vi "Play Sound Effx.vi"(7 "event":enum16{"Play", "Stop"}(ring), 8 "error in (no error)":errorcluster, 9 "path":path, 10 "Sound Effect Off":T1, 11 "Sounds In":T3(array[cluster]) {"Task ID" format="%.0x"}) -> (0 "error out":errorcluster, 3 "Sounds Out":T3(array[cluster]) {"Task ID" format="%.0x"})   [LabVIEW 2021]
uses:
  Typedefs/Sound Effects.ctl
  <vilib>/sound2/lvsound2.llb/Sound Output Task ID.ctl
  <vilib>/sound2/lvsound2.llb/Sound Output Set Volume (Single).vi
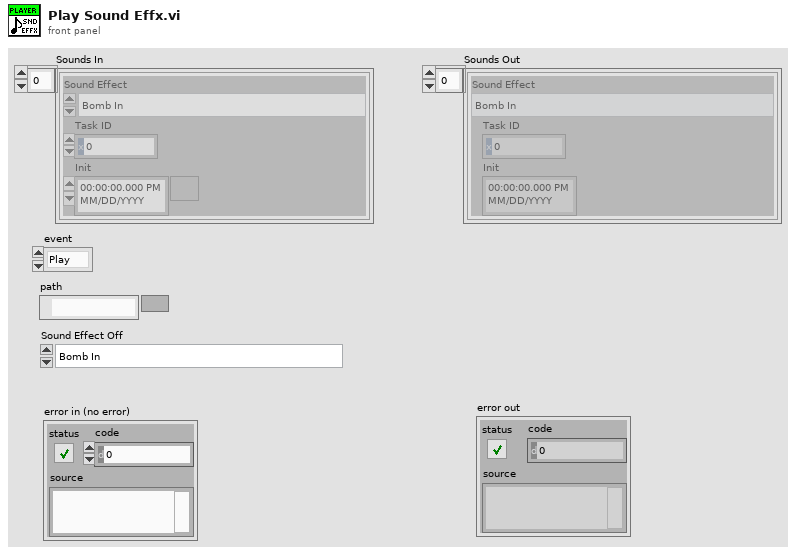
[diagram p1: front panel]
types:
  T1 = typedef "Sound Effects.ctl" = enum16{"Bomb In", "Bomb Out", "Bomb Touched", "Game Over", "Victory", "Eat", "10 Fruits", "Eat2", "Eat3", "Eat4", "MaxShield", "Shield", "10p", "Grape In", "Grape Out", "20p", "30p", "40p", "50p", "60p", "70p", "80p", "90p", "100p", "All shields cracked", "Mouse In", "Mouse Out", "Mouse Eaten", "Grape Eaten", "States Recover", "Broken Shield", "Bonus", "Happy Time", "explode", "Game over musica", "Back Music", "Shield Catch", "Evil lough", "Cricket In", "Cricket eaten", "Lets Go", "Jump1", "Jump2", "Jump3", "Unstoppable", "Troll Music", "winner"}
  T2 = typedef "Sound Output Task ID.ctl" = u32
  T3 = cluster{"Sound Effect":T1, "Task ID":T2, "Init":timestamp}[]
  T4 = cluster{"Sound Effect":T1, "Task ID":T2, "Init":timestamp}
  T5 = cluster{"Sound Effect Off":T1, "task ID":T2, "seconds since 1Jan1904":timestamp}
  T6 = cluster{"Sound Effect Off":T1, "task ID":T2, "seconds since 1Jan1904":timestamp}[]
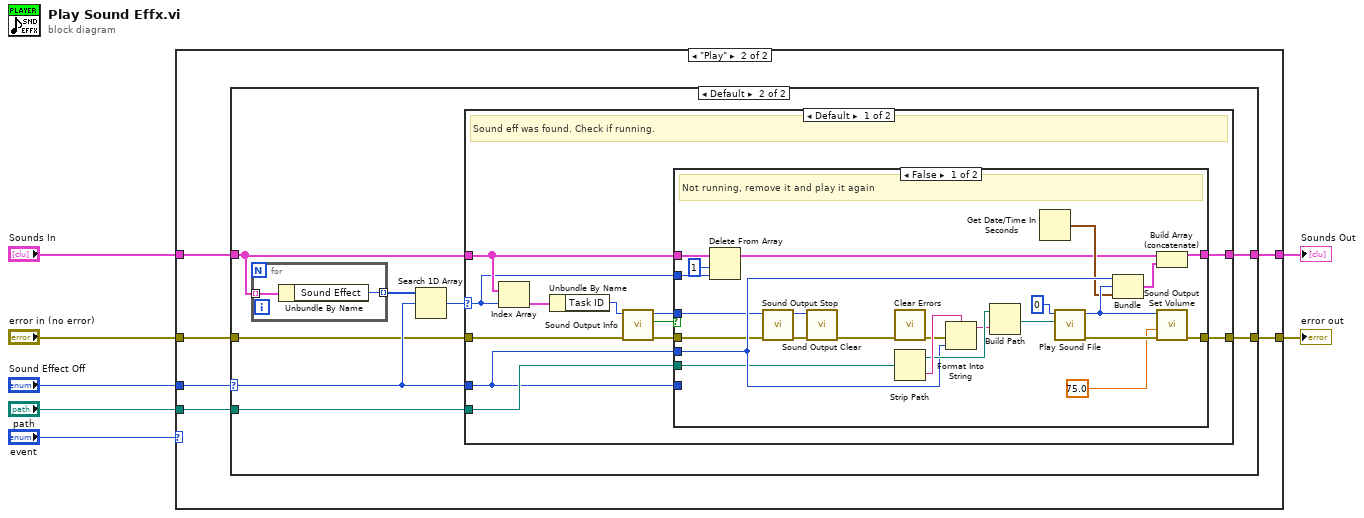
[diagram p0: block diagram]
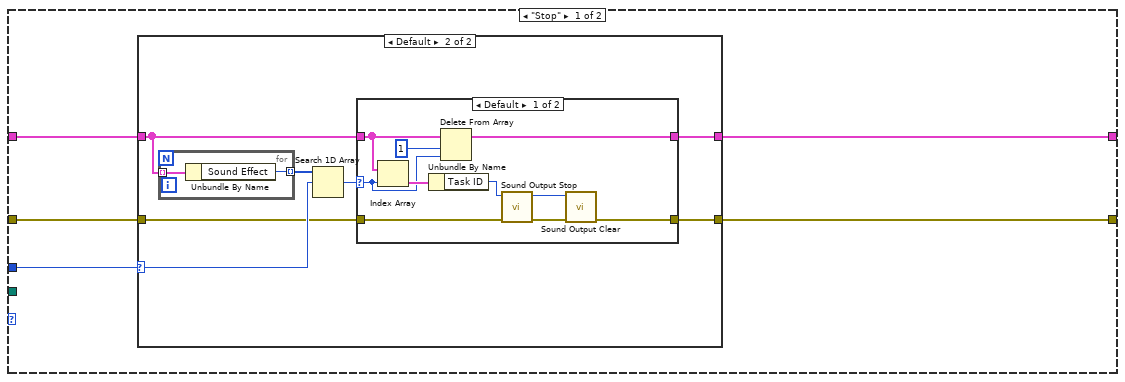
[diagram p2: hidden frame]
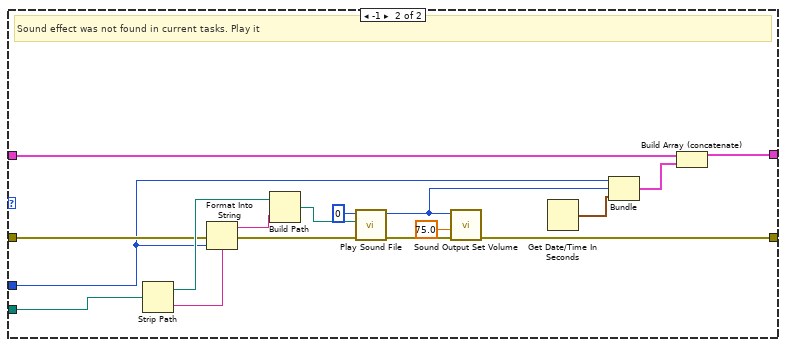
[diagram p7: hidden frame]
diagram:
  n1 = case shown="\"Play\"" "event" {
    tunnel: [w12 w41] -> w7
    tunnel: "Sounds In" -> [w11 w40]
    tunnel: "Sound Effect Off" -> [w10 w39]
    tunnel: "path" -> [_ w38]
    tunnel: [w8 w37] -> w1
    tunnel: "error in (no error)" -> [w9 w36]
    frame "Stop" {
      n2 = case shown="Default" w10 {
        selector: w10 -> [_ w21]
        tunnel: w11 -> [w14 w18]
        tunnel: [w14 w17] -> w12
        tunnel: w9 -> [w13 w16]
        tunnel: [w13 w15] -> w8
        frame "Back Music" {
        }
        frame Default {
          n3 = for {
            tunnel: w18 -> [w35] mode=indexing
            tunnel: [w34] -> w20 mode=indexing
            n4 = Unbundle By Name(w35) -> ("Sound Effect"=w34:T1)
          }
          n5 = Search 1D Array(1D array=w20, element=w21) -> (index of element=w19:i32)  [unwired: 1 in]
          n6 = case shown="Default" w19 {
            selector: w19 -> [w25 _]
            tunnel: w18 -> [w27 w33]
            tunnel: [w24 w33] -> w17
            tunnel: w16 -> [w23 w32]
            tunnel: [w22 w32] -> w15
            frame Default {
              n7 = Index Array(array=w27, index=w25) -> (element=w31:T4)
              n8 = Unbundle By Name(w31) -> ("Task ID"=w30:T2)
              n9 = Delete From Array(array=w27, length=1, index=w25) -> (array with subset deleted=w24:T3)  [unwired: 1 out]
              n10 = call <vilib>:"Sound Output Stop.vi"("error in (no error)"=w23, "task ID"=w30) -> ("error out"=w28:errorcluster, "task ID out"=w29:T2)  [unwired: 8 in]
              n11 = call <vilib>:"Sound Output Clear.vi"("error in (no error)"=w28, "task ID"=w29) -> ("error out"=w22:errorcluster)  [unwired: 9 in]
            }
            frame -1 {
            }
          }
        }
      }
    }
    frame "Play" {
      n12 = case shown="Default" w39 {
        selector: w39 -> [_ w47]
        tunnel: w40 -> [w43 w49]
        tunnel: [w43 w48] -> w41
        tunnel: w38 -> [_ w46]
        tunnel: [w42 w45] -> w37
        tunnel: w36 -> [w42 w44]
        frame "Back Music" {
        }
        frame Default {
          n13 = for {
            tunnel: w49 -> [w108] mode=indexing
            tunnel: [w107] -> w51 mode=indexing
            n14 = Unbundle By Name(w108) -> ("Sound Effect"=w107:T1)
          }
          n15 = Search 1D Array(1D array=w51, element=w47) -> (index of element=w50:i32)  [unwired: 1 in]
          n16 = case shown="Default" w50 {
            selector: w50 -> [w52 _]
            tunnel: w49 -> [w60 w98]
            tunnel: [w59 w97] -> w48
            tunnel: w47 -> [w53 w92]
            tunnel: w46 -> [w56 w96]
            tunnel: [w55 w95] -> w45
            tunnel: w44 -> [w54 w94]
            frame Default {
              # "Sound eff was found. Check if running."
              n17 = Index Array(array=w60, index=w52) -> (element=w63:T4)
              n18 = Unbundle By Name(w63) -> ("Task ID"=w62:T2)
              n19 = call <vilib>:"Sound Output Info.vi"("error in (no error)"=w54, "task ID"=w62) -> ("error out"=w57:errorcluster, "is playing?"=w61:bool, "task ID out"=w58:T2)  [unwired: 6 in, 1 out]
              n20 = case shown="False" w61 {
                tunnel: w60 -> [w80 w89]
                tunnel: [w79 w89] -> w59
                tunnel: w58 -> [w73 _]
                tunnel: w57 -> [w72 w88]
                tunnel: w53 -> [w77 _]
                tunnel: w56 -> [w76 _]
                tunnel: [w70 w88] -> w55
                tunnel: w53 -> [_ _]
                tunnel: w52 -> [w65 _]
                frame False {
                  # "Not running, remove it and play it again"
                  n21 = Delete From Array(array=w80, length=1, index=w65) -> (array with subset deleted=w66:T3)  [unwired: 1 out]
                  n22 = call <vilib>:"Sound Output Stop.vi"("error in (no error)"=w72, "task ID"=w73) -> ("error out"=w74:errorcluster, "task ID out"=w75:T2)  [unwired: 8 in]
                  n23 = call <vilib>:"Sound Output Clear.vi"("error in (no error)"=w74, "task ID"=w75) -> ("error out"=w71:errorcluster)  [unwired: 9 in]
                  n24 = call <vilib>:"Clear Errors.vi"("error in (no error)"=w71) -> ("error out"=w69:errorcluster)  [unwired: 5 in, 1 out]
                  n25 = Strip Path(path=w76) -> (stripped path=w84:path, name=w85:string)
                  n26 = Format Into String(format string=w85, error in=w69, w77) -> (resulting string=w83:string)  [unwired: 1 in, 1 out]
                  n27 = Build Path(base path=w84, name or relative path=w83) -> (appended path=w82:path)
                  n28 = Get Date/Time In Seconds() -> (seconds since 1Jan1904=w67:timestamp)
                  n29 = call <vilib>:"Play Sound File.vi"("path"=w82, "device ID"=u32 0) -> ("error out"=w86:errorcluster, "task ID"=w81:T2)  [unwired: 8 in]
                  n30 = Bundle("Sound Effect Off"=w77, "task ID"=w81, "seconds since 1Jan1904"=w67) -> (w78:T5)  [unwired: 1 in]
                  n31 = Build Array (concatenate)(w66, w78) -> (w79:T6)
                  n32 = call-poly <vilib>:"Sound Output Set Volume.vi"("error in (no error)"=w86, "volume"=75.0, "task ID"=w81) -> ("error out"=w70:errorcluster)  [unwired: 7 in, 1 out]
                }
                frame True {
                  # "Is playing, ignore event"
                }
              }
            }
            frame -1 {
              # "Sound effect was not found in current tasks. Play it"
              n33 = Strip Path(path=w96) -> (stripped path=w102:path, name=w103:string)
              n34 = Format Into String(format string=w103, error in=w94, w92) -> (resulting string=w101:string, error out=w93:errorcluster)  [unwired: 1 in]
              n35 = Build Path(base path=w102, name or relative path=w101) -> (appended path=w91:path)
              n36 = call <vilib>:"Play Sound File.vi"("error in (no error)"=w93, "path"=w91, "device ID"=u32 0) -> ("error out"=w105:errorcluster, "task ID"=w100:T2)  [unwired: 7 in]
              n37 = call-poly <vilib>:"Sound Output Set Volume.vi"("error in (no error)"=w105, "volume"=75.0, "task ID"=w100) -> ("error out"=w95:errorcluster)  [unwired: 7 in, 1 out]
              n38 = Get Date/Time In Seconds() -> (seconds since 1Jan1904=w90:timestamp)
              n39 = Bundle("Sound Effect Off"=w92, "task ID"=w100, "seconds since 1Jan1904"=w90) -> (w99:T5)  [unwired: 1 in]
              n40 = Build Array (concatenate)(w98, w99) -> (w97:T6)
            }
          }
        }
      }
    }
  }
  "Sounds Out" <- w7
  "error out" <- w1
